vi "Activate Subscription Policy.vi"(8 "error in (no error)":errorcluster, 11 "Subscription Policy":T1) -> (0 "error out":errorcluster)   [LabVIEW 2017, in "IMediator.lvlib" / "ISubscriptionPolicy.lvclass"]
doc: "This method decides whether or not to send or otherwise handle the new data value. The policy is set and maintained by the subscriber. The Topic Actor knows no policy details, it just passes the new value in. If there is a failure inside this method, the Topic Actor must assume the listener is no longer valid (dead/unrecoverable) and should delete it from the Subscriber list.\n\n<License>\nCopyright © 2017 Composed Systems, LLC | All rights reserved\nwww.composed.io\n\nAuthor: Ethan Stern <ethan.stern@composed.io>\n\nThis software is provided \"AS IS\" WITHOUT WARRANTIES, either express or implied, AND IS FOR EDUCATIONAL PURPOSES ONLY.\n</License>"
uses:
  <vilib>/gpm_packages/@cs/mva-core/Source/IMediator/ISubscriptionPolicy/ISubscriptionPolicy.lvclass
  <vilib>/gpm_packages/@cs/mva-core/Source/IMediator/ISubscriptionPolicy/ISubscriptionPolicy Reference.ctl
  <vilib>/gpm_packages/@cs/mva-core/Source/IMediator/ISubscriptionPolicy/ISubscriptionPolicy.lvclass/ISubscriptionPolicy.ctl
panel:
  out "Subscription Policy Out":T1
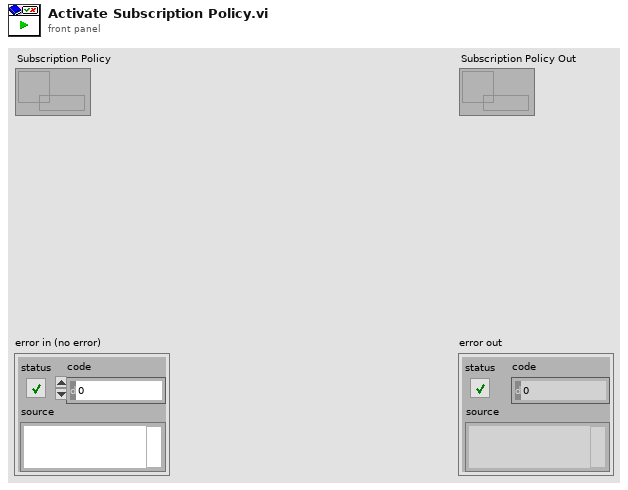
[diagram p1: front panel]
types:
  T1 = typedef "IMediator.lvlib/ISubscriptionPolicy.lvclass/ISubscriptionPolicy Reference.ctl" = refnum<data-value>
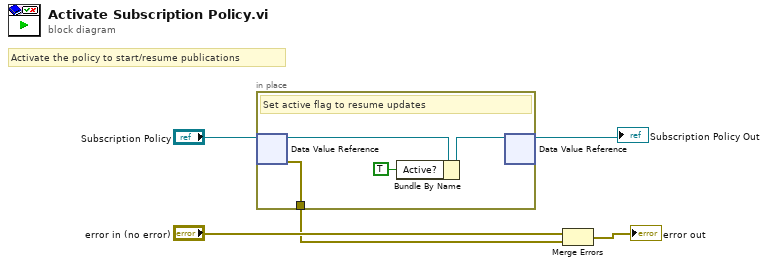
[diagram p0: block diagram]
diagram:
  # "Activate the policy to start/resume publications"
  n1 = in-place {
    in-place-border: [w8] -> w2
    # "Set active flag to resume updates"
    n2 = in-place-dvr #1("Subscription Policy") -> (w9:refnum<class "ISubscriptionPolicy.lvclass">, w8:errorcluster)
    n3 = Bundle By Name(cluster=w9, "Active?"=TRUE) -> (w7:refnum<class "ISubscriptionPolicy.lvclass">)
    n4 = in-place-dvr #1(w7) -> (→"Subscription Policy Out":T1)  [unwired: 1 out]
  }
  n5 = Merge Errors("error in (no error)", w2) -> (→"error out":errorcluster)
